vi "ESP301_StandAlone.vi"(0 "COM_PORT":string="COM13", 5 "stop":bool, 9 "SONDE_IN":bool) -> (3 "ESP301_ROT_MO":bool, 4 "ROT_mouvement":bool, 6 "ESP301_ROT_POS":dbl=3395.0 caption="Relacher pour \nmodifier TCS" format="%.2f", 8 "BRAS_OUT":bool, 10 "ESP301_BRAS_POS":dbl=3395.0 caption="Relacher pour \nmodifier TCS" format="%.2f", 14 "ESP301_BRAS_MO":bool, 15 "BRAS _mouvement":bool)   [LabVIEW 2019]
panel:
  in  "Reconnecter":bool
  in  "ROT_NORD_Value":dbl=120.0
  in  "BRAS_OUT_Value":dbl=40.0
  in  "BRAS_IN_Value":dbl=-6.0
  in  "BRAS_Target":dbl=30.0
  in  "BRAS_state":u16(ring) items=["Error"=6, "Stop"=5, "Out"=4, "In"=3, "Set"=2, "Home"=1, "Standby"=0]
  out "Comm":bool
  in  "ROT_Target":dbl=30.0
  in  "ROT_state":u16(ring) items=["Error"=6, "Stop"=4, "Nord"=3, "Set"=2, "Home"=1, "Standby"=0]
  in  "ESP301_BRAS_STOP":bool caption="À la cible"
  in  "ESP301_BRAS_SET":bool caption="À la cible"
  in  "ESP301_BRAS_OUT":bool caption="À la cible"
  in  "ESP301_BRAS_IN":bool caption="À la cible"
  in  "ESP301_BRAS_HOME":bool caption="À la cible"
  in  "ESP301_ROT_STOP":bool caption="À la cible"
  in  "ESP301_ROT_SET":bool caption="À la cible"
  in  "ESP301_ROT_NORD":bool caption="À la cible"
  in  "ESP301_ROT_HOME":bool caption="À la cible"
  # "Rotateur Pesto"
  # "Bras  Pesto"
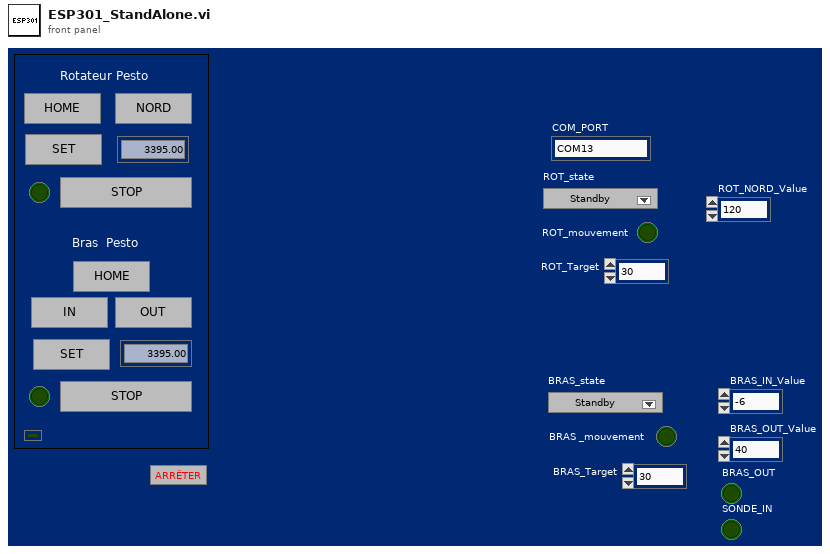
[diagram p1: front panel]
types:
  T1 = enum8{"Enabled", "Disabled", "Disabled and Grayed Out"}
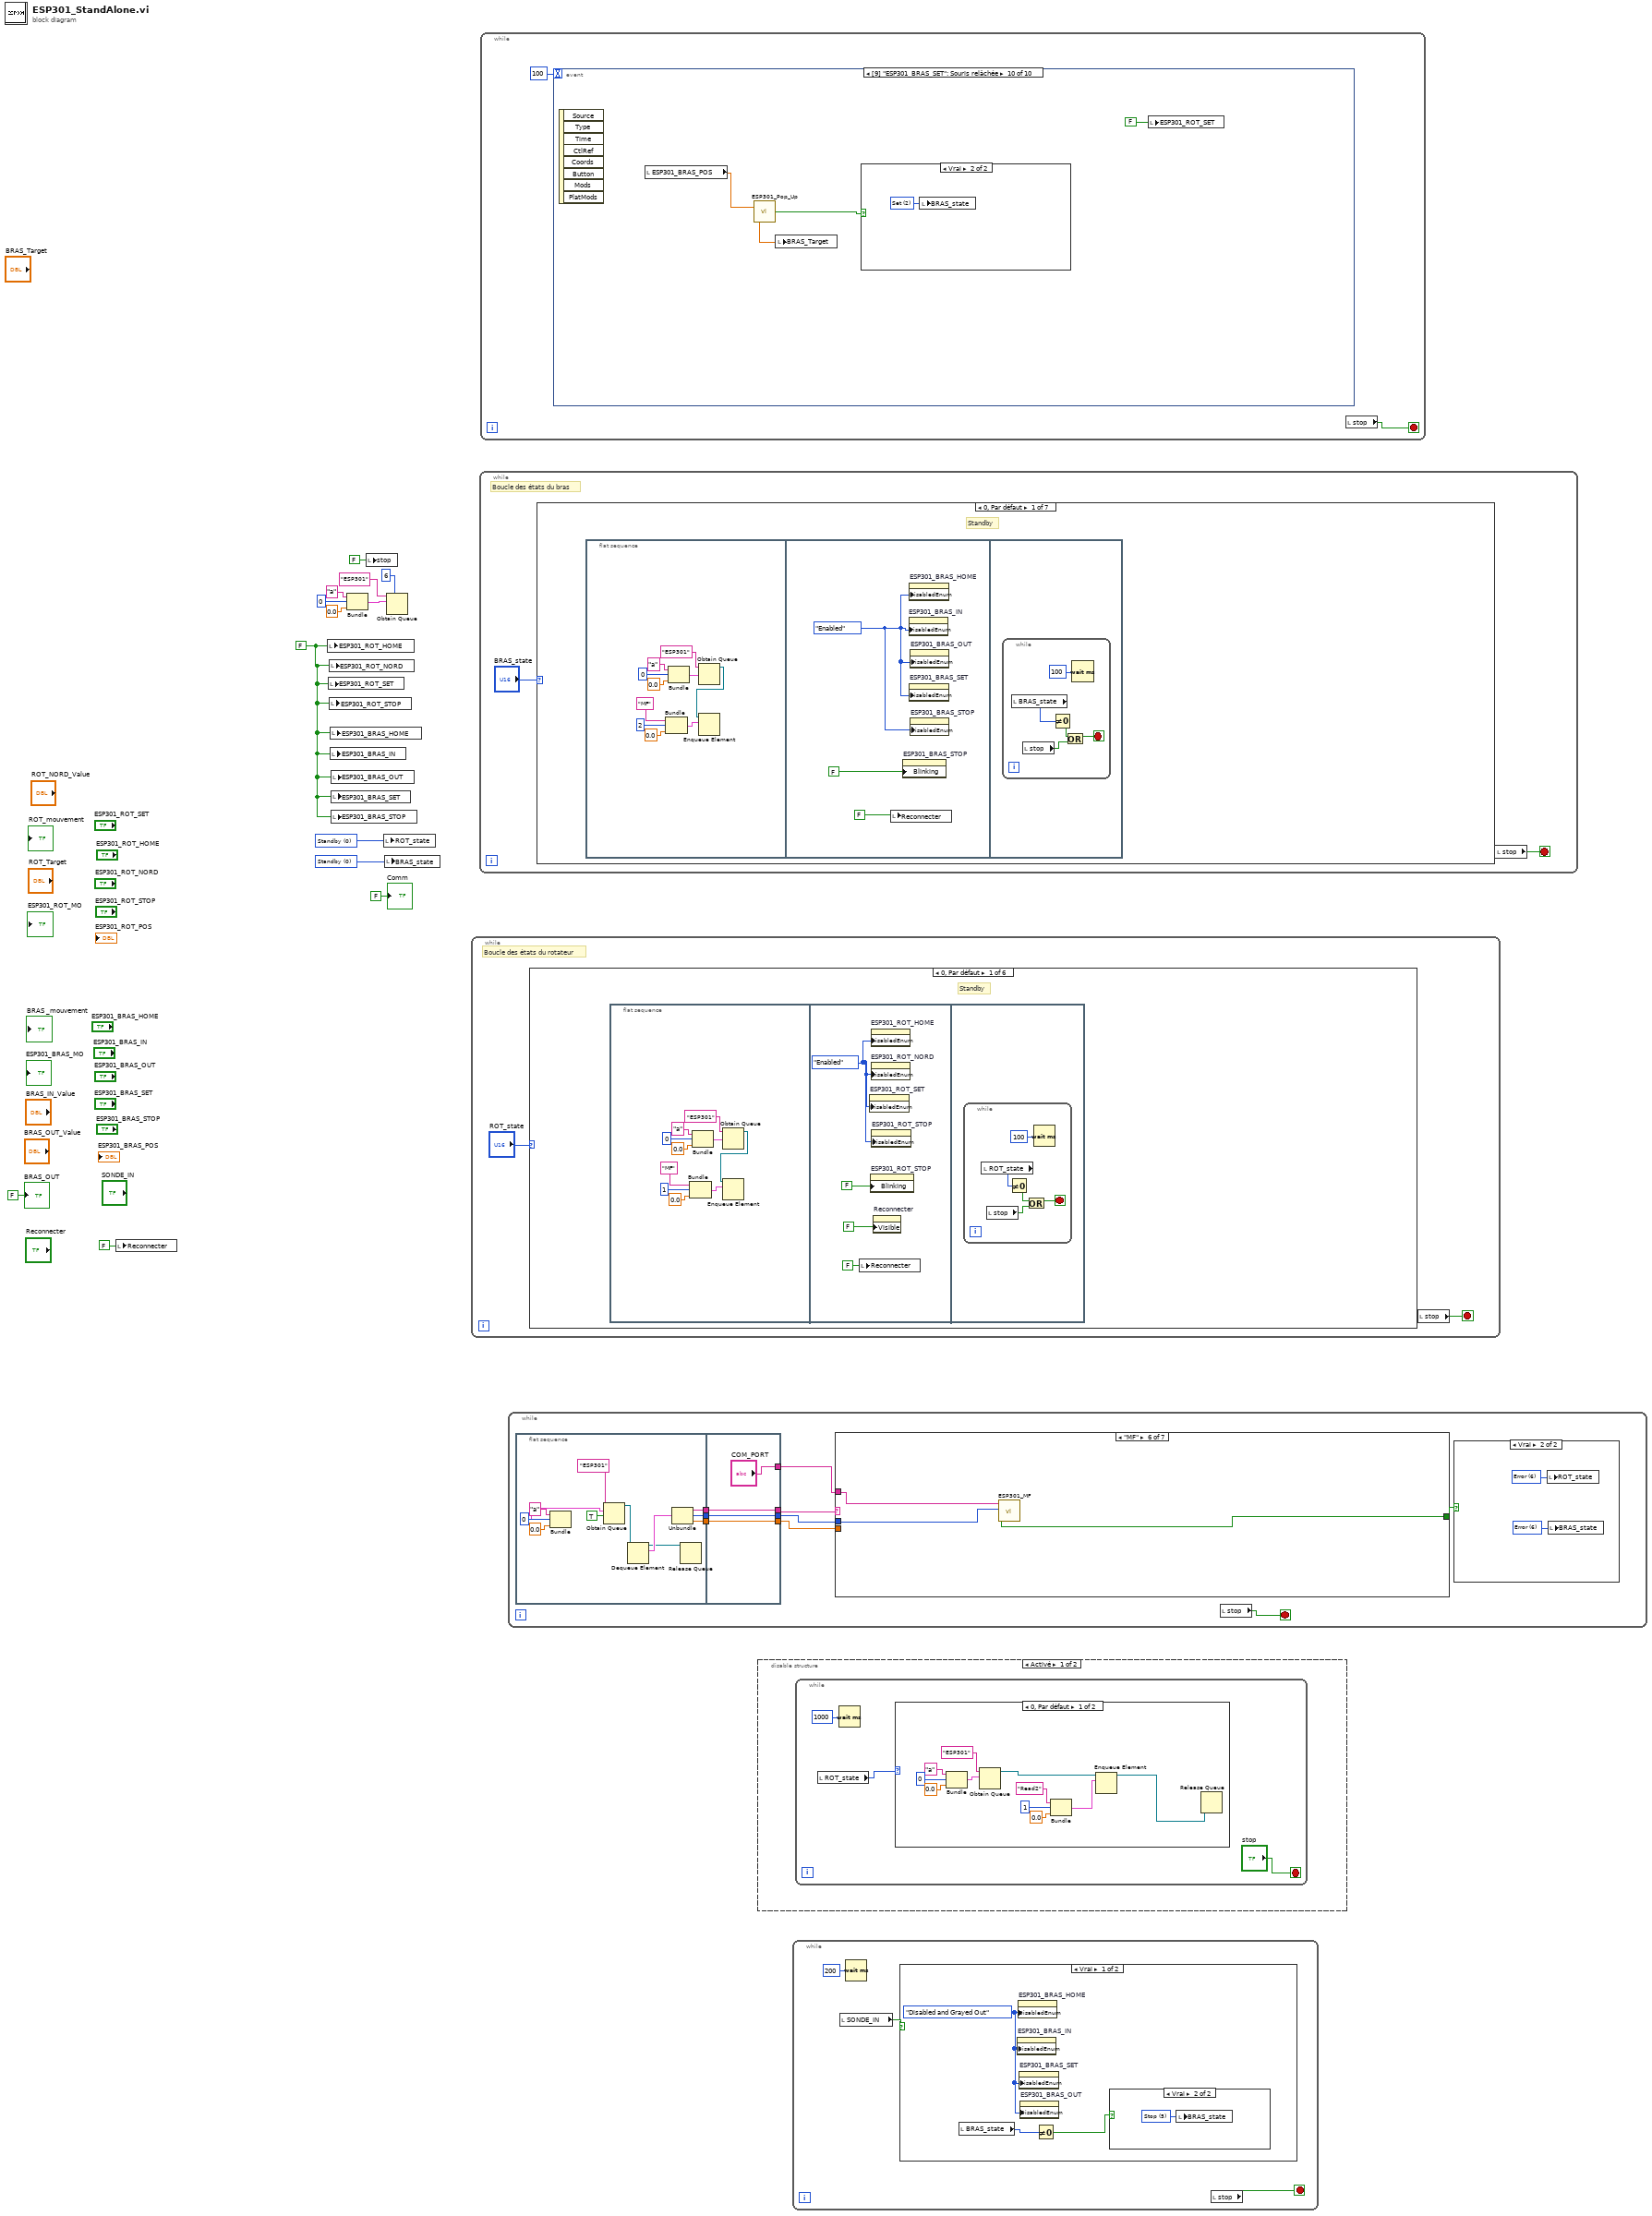
[diagram p0: block diagram]
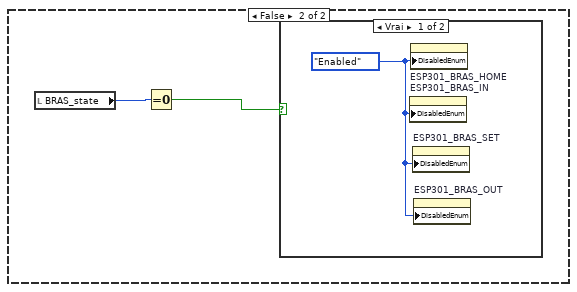
[diagram p3: hidden frame]
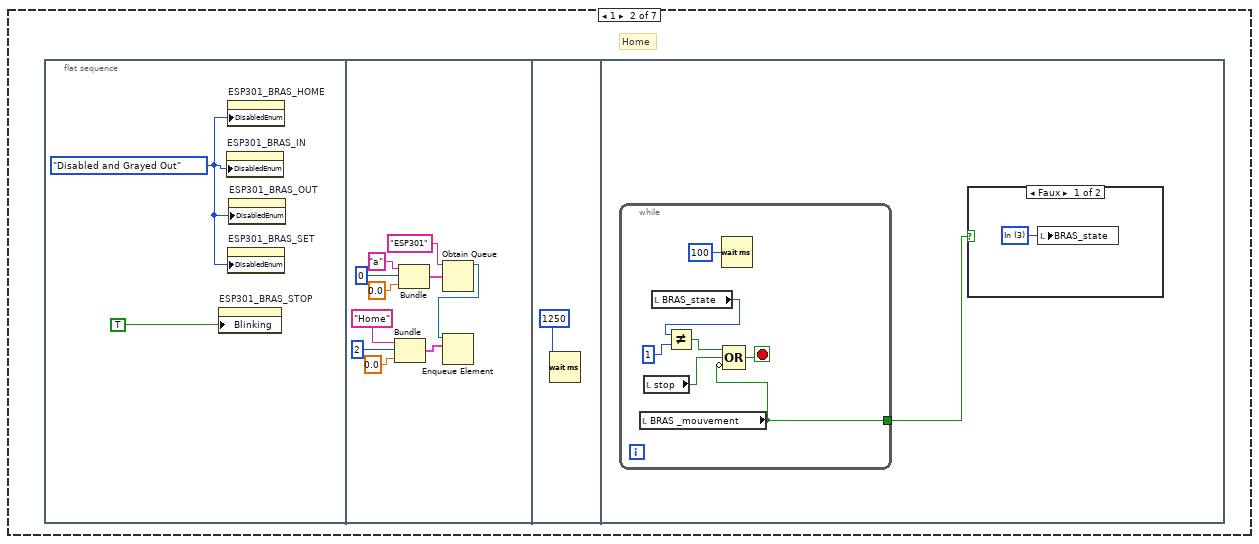
[diagram p5: hidden frame]
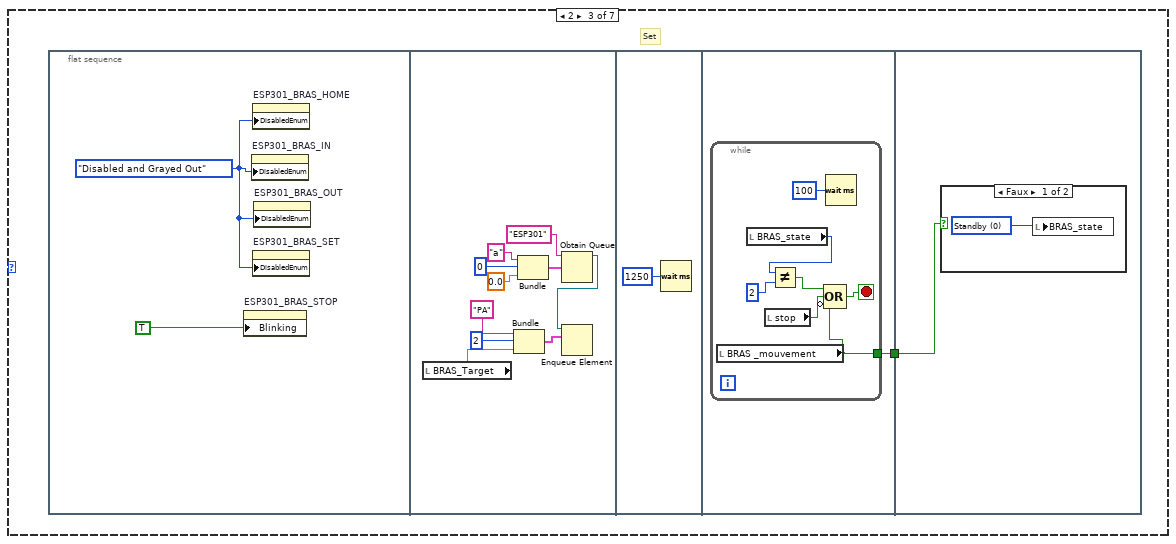
[diagram p7: hidden frame]
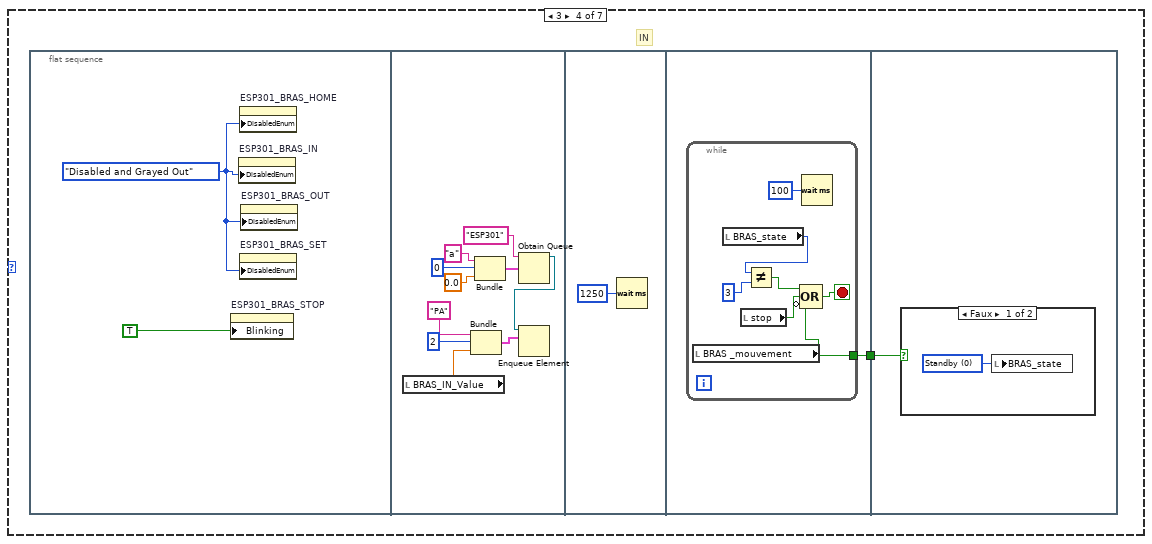
[diagram p9: hidden frame]
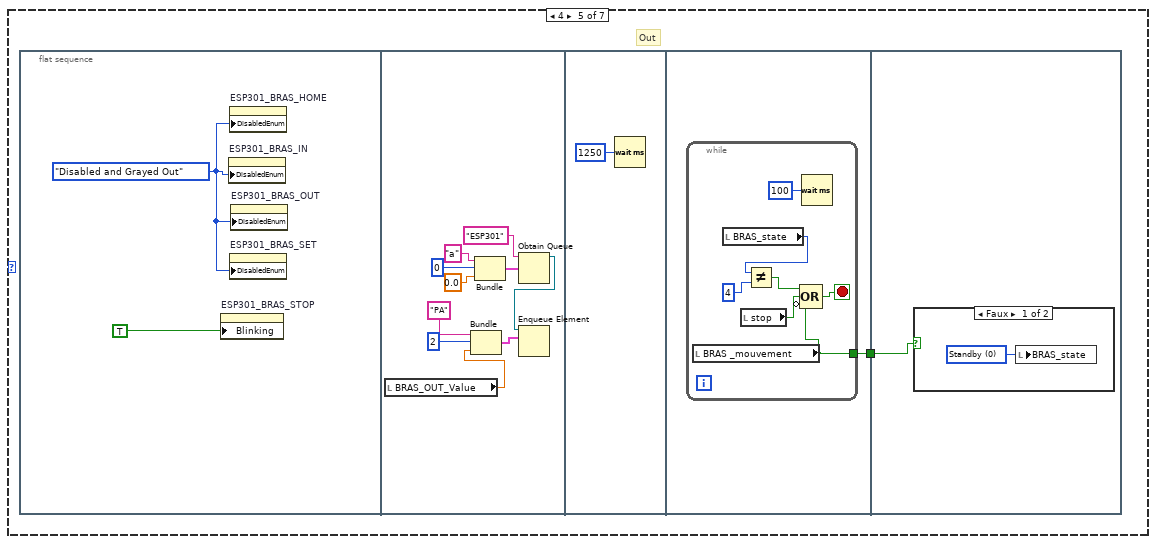
[diagram p11: hidden frame]
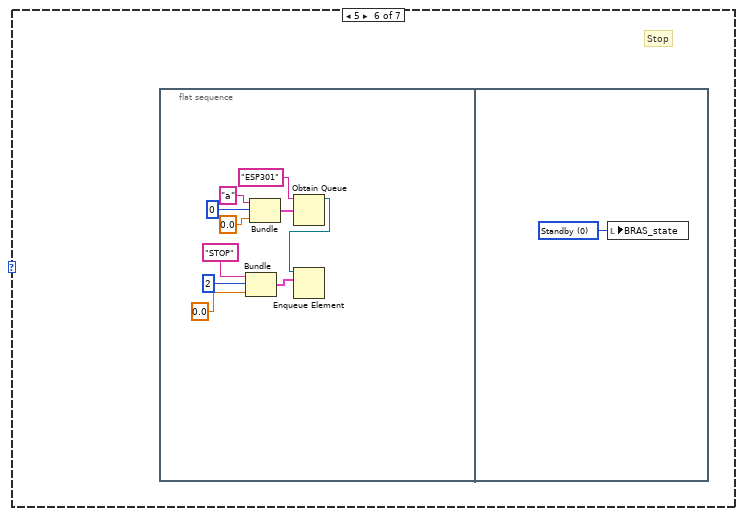
[diagram p13: hidden frame]
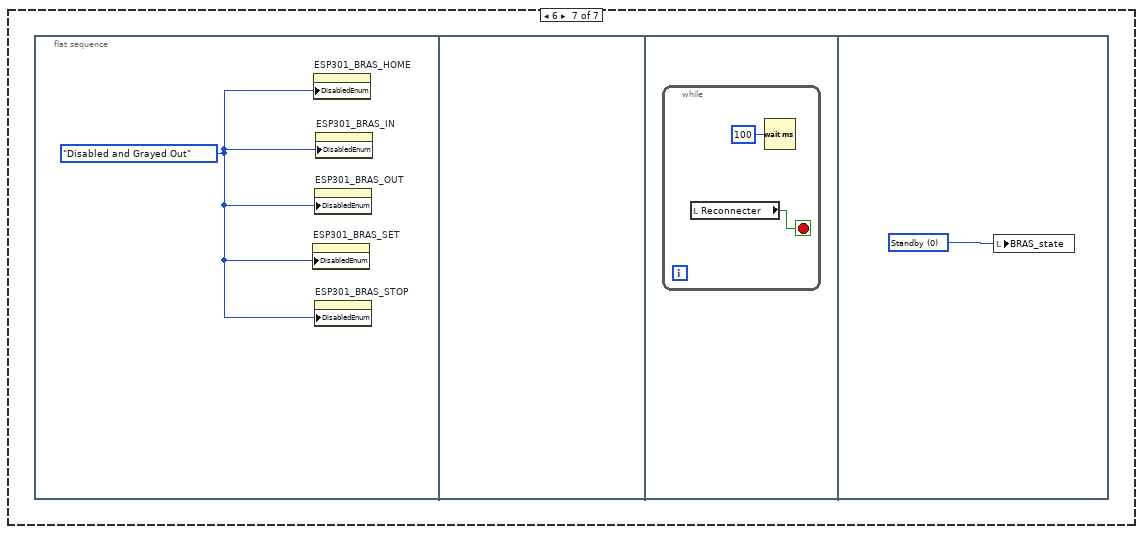
[diagram p14: hidden frame]
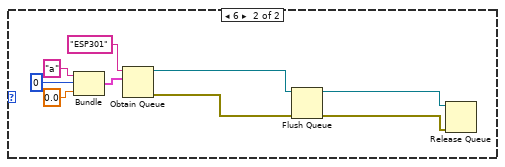
[diagram p15: hidden frame]
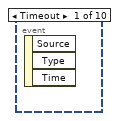
[diagram p17: hidden frame]
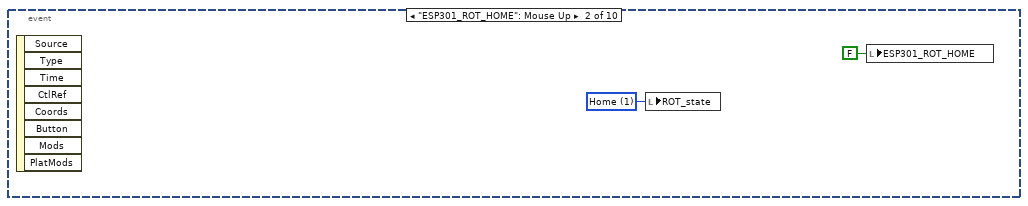
[diagram p18: hidden frame]
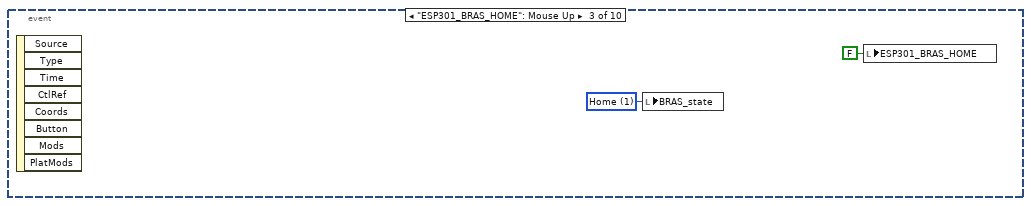
[diagram p19: hidden frame]
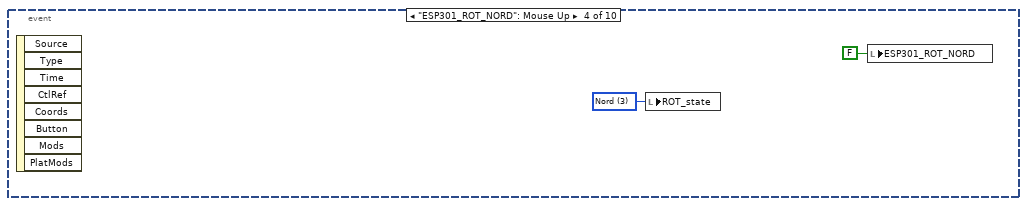
[diagram p20: hidden frame]
diagram:
  w4 = u16 0 items=["Stop"=4, "Nord"=3, "Set"=2, "Home"=1, "Standby"=0] ("BRAS_state")
  w5 = FALSE ("ESP301_ROT_HOME")
  w7 = u16 0 items=["Go"=2, "Home"=1, "Standby"=0] ("Rotateur_state")
  n1 = local write "Reconnecter"(FALSE ("Reconnecter")) -> ()
  n2 = local write "ESP301_ROT_HOME"(w5) -> ()
  n3 = local write "ESP301_ROT_SET"(w5) -> ()
  n4 = local write "ESP301_ROT_NORD"(w5) -> ()
  n5 = local write "ESP301_ROT_STOP"(w5) -> ()
  n6 = local write "ESP301_BRAS_HOME"(w5) -> ()
  n7 = local write "ESP301_BRAS_IN"(w5) -> ()
  n8 = local write "ESP301_BRAS_OUT"(w5) -> ()
  n9 = local write "ESP301_BRAS_SET"(w5) -> ()
  n10 = local write "ESP301_BRAS_STOP"(w5) -> ()
  n11 = Bundle("a", 0, 0.0) -> (w11:cluster{string, i32, dbl})  [unwired: 1 in]
  n12 = local write "stop"(FALSE ("stop")) -> ()
  n13 = local write "ROT_state"(w7) -> ()
  n14 = local write "BRAS_state"(w4) -> ()
  n15 = Obtain Queue(max queue size (-1, unlimited)=6 ("taille max de la file d'attente (-1, non limitée)"), name (unnamed)="ESP301" ("nom (aucun)"), element data type=w11) -> ()  [unwired: 2 in, 3 out]
  n16 = while {
    stop <- w15 stop-if-true
    # "Boucle des états du rotateur"
    n17 = case shown="0, Par défaut" "ROT_state" {
      frame 0, Default {
        # "Standby"
        n18 = flat-sequence {
          frame #0 {
            n19 = Bundle("MF", 1, 0.0) -> (w17:cluster{string, i32, dbl})  [unwired: 1 in]
            n20 = Bundle("a", 0, 0.0) -> (w23:cluster{string, i32, dbl})  [unwired: 1 in]
            n21 = Obtain Queue(name (unnamed)="ESP301" ("nom (aucun)"), element data type=w23) -> (queue out=w21:refnum<queue>)  [unwired: 3 in, 2 out]
            n22 = Enqueue Element(queue=w21, element=w17) -> ()  [unwired: 2 in, 3 out]
          }
          frame #1 {
            w27 = T1."Enabled" ("Désactivé")
            n23 = local write "Reconnecter"(FALSE ("Reconnecter")) -> ()
            n24 = property on="ESP301_ROT_SET" class="Bool (strict)"("DisabledEnum"=w27) -> ()  [unwired: 2 in, 2 out]
            n25 = property on="ESP301_ROT_STOP" class="Bool (strict)"("Blinking"=FALSE ("Clignotant")) -> ()  [unwired: 2 in, 2 out]
            n26 = property on="ESP301_ROT_HOME" class="Bool (strict)"("DisabledEnum"=w27) -> ()  [unwired: 2 in, 2 out]
            n27 = property on="ESP301_ROT_NORD" class="Bool (strict)"("DisabledEnum"=w27) -> ()  [unwired: 2 in, 2 out]
            n28 = property on="ESP301_ROT_STOP" class="Bool (strict)"("DisabledEnum"=w27) -> ()  [unwired: 2 in, 2 out]
            n29 = property on="Reconnecter" class="Bool (strict)"("Visible"=FALSE) -> ()  [unwired: 2 in, 2 out]
          }
          frame #2 {
            n30 = while {
              stop <- w32 stop-if-true
              n31 = local read "ROT_state"() -> (w34:u16)
              n32 = local read "stop"() -> (w31:bool)
              n33 = Not Equal To 0?(x=w34) -> (x != 0?=w30:bool)
              n34 = Or(x=w30, y=w31) -> (x .or. y?=w32:bool)
              n35 = Wait (ms)(milliseconds to wait=u32 100 ("attente (ms)")) -> ()  [unwired: 1 out]
            }
          }
        }
      }
      frame 1 {
        # "Home"
        n36 = flat-sequence {
          tunnel: [w49] -> w35
          tunnel: w35 -> [w57]
          frame #0 {
            w36 = T1."Disabled and Grayed Out" ("Désactivé")
            n37 = property on="ESP301_ROT_SET" class="Bool (strict)"("DisabledEnum"=w36) -> ()  [unwired: 2 in, 2 out]
            n38 = property on="ESP301_ROT_STOP" class="Bool (strict)"("Blinking"=TRUE ("Clignotant")) -> ()  [unwired: 2 in, 2 out]
            n39 = property on="ESP301_ROT_HOME" class="Bool (strict)"("DisabledEnum"=w36) -> ()  [unwired: 2 in, 2 out]
            n40 = property on="ESP301_ROT_NORD" class="Bool (strict)"("DisabledEnum"=w36) -> ()  [unwired: 2 in, 2 out]
          }
          frame #1 {
            n41 = local read "ROT_NORD_Value"() -> (w38:dbl)
            n42 = Bundle("Home", 1, "ROT_NORD_Value"=w38) -> (w40:cluster{string, i32, "ROT_NORD_Value":dbl})  [unwired: 1 in]
            n43 = Bundle("a", 0, 0.0) -> (w45:cluster{string, i32, dbl})  [unwired: 1 in]
            n44 = Obtain Queue(name (unnamed)="ESP301" ("nom (aucun)"), element data type=w45) -> (queue out=w43:refnum<queue>)  [unwired: 3 in, 2 out]
            n45 = Enqueue Element(queue=w43, element=w40) -> ()  [unwired: 2 in, 3 out]
          }
          frame #2 {
            n46 = Wait (ms)(milliseconds to wait=u32 1250 ("attente (ms)")) -> ()  [unwired: 1 out]
          }
          frame #3 {
            n47 = while {
              tunnel: [w50] -> w49
              stop <- w53 stop-if-true
              n48 = local read "stop"() -> (w51:bool)
              n49 = local read "ROT_state"() -> (w55:u16)
              n50 = local read "ROT_mouvement"() -> (w50:bool)
              n51 = Not Equal?(x=w55, y=u16 1) -> (x != y?=w52:bool)
              n52 = Wait (ms)(milliseconds to wait=u32 100 ("attente (ms)")) -> ()  [unwired: 1 out]
              n53 = Compound Arithmetic op=OR ("Opérateur arithmétique")(w52, w51, invert w50) -> (w53:bool)
            }
          }
          frame #4 {
            n54 = case shown="Faux" w57 {
              frame False {
                w58 = u16 3 items=["Stop"=4, "Nord"=3, "Set"=2, "Home"=1, "Standby"=0] ("ROT_state")
                n55 = local write "ROT_state"(w58) -> ()
              }
              frame True {
              }
            }
          }
        }
      }
      frame 2 {
        # "Set"
        n56 = flat-sequence {
          tunnel: [w73] -> w59
          tunnel: w59 -> [w81]
          frame #0 {
            w60 = T1."Disabled and Grayed Out" ("Désactivé")
            n57 = property on="ESP301_ROT_SET" class="Bool (strict)"("DisabledEnum"=w60) -> ()  [unwired: 2 in, 2 out]
            n58 = property on="ESP301_ROT_STOP" class="Bool (strict)"("Blinking"=TRUE ("Clignotant")) -> ()  [unwired: 2 in, 2 out]
            n59 = property on="ESP301_ROT_HOME" class="Bool (strict)"("DisabledEnum"=w60) -> ()  [unwired: 2 in, 2 out]
            n60 = property on="ESP301_ROT_NORD" class="Bool (strict)"("DisabledEnum"=w60) -> ()  [unwired: 2 in, 2 out]
          }
          frame #1 {
            n61 = local read "ROT_Target"() -> (w62:dbl)
            n62 = Bundle("PA", 1, "ROT_Target"=w62) -> (w64:cluster{string, i32, "ROT_Target":dbl})  [unwired: 1 in]
            n63 = Bundle("a", 0, 0.0) -> (w69:cluster{string, i32, dbl})  [unwired: 1 in]
            n64 = Obtain Queue(name (unnamed)="ESP301" ("nom (aucun)"), element data type=w69) -> (queue out=w67:refnum<queue>)  [unwired: 3 in, 2 out]
            n65 = Enqueue Element(queue=w67, element=w64) -> ()  [unwired: 2 in, 3 out]
          }
          frame #2 {
            n66 = Wait (ms)(milliseconds to wait=u32 1250 ("attente (ms)")) -> ()  [unwired: 1 out]
          }
          frame #3 {
            n67 = while {
              tunnel: [w74] -> w73
              stop <- w77 stop-if-true
              n68 = local read "ROT_mouvement"() -> (w74:bool)
              n69 = local read "ROT_state"() -> (w79:u16)
              n70 = local read "stop"() -> (w75:bool)
              n71 = Not Equal?(x=w79, y=u16 2) -> (x != y?=w76:bool)
              n72 = Compound Arithmetic op=OR ("Opérateur arithmétique")(w76, w75, invert w74) -> (w77:bool)
              n73 = Wait (ms)(milliseconds to wait=u32 100 ("attente (ms)")) -> ()  [unwired: 1 out]
            }
          }
          frame #4 {
            n74 = case shown="Faux" w81 {
              frame False {
                w82 = u16 0 items=["Nord"=3, "Go"=2, "Home"=1, "Standby"=0] ("ROT_state")
                n75 = local write "ROT_state"(w82) -> ()
              }
              frame True {
              }
            }
          }
        }
      }
      frame 3 {
        # "Nord"
        n76 = flat-sequence {
          tunnel: [w97] -> w83
          tunnel: w83 -> [w105]
          frame #0 {
            w84 = T1."Disabled and Grayed Out" ("Désactivé")
            n77 = property on="ESP301_ROT_SET" class="Bool (strict)"("DisabledEnum"=w84) -> ()  [unwired: 2 in, 2 out]
            n78 = property on="ESP301_ROT_STOP" class="Bool (strict)"("Blinking"=TRUE ("Clignotant")) -> ()  [unwired: 2 in, 2 out]
            n79 = property on="ESP301_ROT_HOME" class="Bool (strict)"("DisabledEnum"=w84) -> ()  [unwired: 2 in, 2 out]
            n80 = property on="ESP301_ROT_NORD" class="Bool (strict)"("DisabledEnum"=w84) -> ()  [unwired: 2 in, 2 out]
          }
          frame #1 {
            n81 = Bundle("PA", 1, 0.0) -> (w88:cluster{string, i32, dbl})  [unwired: 1 in]
            n82 = Bundle("a", 0, 0.0) -> (w93:cluster{string, i32, dbl})  [unwired: 1 in]
            n83 = Obtain Queue(name (unnamed)="ESP301" ("nom (aucun)"), element data type=w93) -> (queue out=w91:refnum<queue>)  [unwired: 3 in, 2 out]
            n84 = Enqueue Element(queue=w91, element=w88) -> ()  [unwired: 2 in, 3 out]
          }
          frame #2 {
            n85 = Wait (ms)(milliseconds to wait=u32 1250 ("attente (ms)")) -> ()  [unwired: 1 out]
          }
          frame #3 {
            n86 = while {
              tunnel: [w98] -> w97
              stop <- w101 stop-if-true
              n87 = local read "ROT_mouvement"() -> (w98:bool)
              n88 = local read "ROT_state"() -> (w103:u16)
              n89 = local read "stop"() -> (w99:bool)
              n90 = Not Equal?(x=w103, y=u16 3) -> (x != y?=w100:bool)
              n91 = Compound Arithmetic op=OR ("Opérateur arithmétique")(w100, w99, invert w98) -> (w101:bool)
              n92 = Wait (ms)(milliseconds to wait=u32 100 ("attente (ms)")) -> ()  [unwired: 1 out]
            }
          }
          frame #4 {
            n93 = case shown="Faux" w105 {
              frame False {
                w106 = u16 0 items=["Nord"=3, "Go"=2, "Home"=1, "Standby"=0] ("ROT_state")
                n94 = local write "ROT_state"(w106) -> ()
              }
              frame True {
              }
            }
          }
        }
      }
      frame 4 {
        # "Stop"
        n95 = flat-sequence {
          frame #0 {
            n96 = Bundle("STOP", 1, 0.0) -> (w109:cluster{string, i32, dbl})  [unwired: 1 in]
            n97 = Bundle("a", 0, 0.0) -> (w114:cluster{string, i32, dbl})  [unwired: 1 in]
            n98 = Obtain Queue(name (unnamed)="ESP301" ("nom (aucun)"), element data type=w114) -> (queue out=w112:refnum<queue>)  [unwired: 3 in, 2 out]
            n99 = Enqueue Element(queue=w112, element=w109) -> ()  [unwired: 2 in, 3 out]
          }
          frame #1 {
            w117 = u16 0 items=["Stop"=4, "Nord"=3, "Set"=2, "Home"=1, "Standby"=0] ("ROT_state")
            n100 = local write "ROT_state"(w117) -> ()
          }
        }
      }
      frame 6 {
        # "ERROR"
        n101 = flat-sequence {
          frame #0 {
            w119 = T1."Disabled and Grayed Out" ("Désactivé")
            n102 = property on="ESP301_ROT_SET" class="Bool (strict)"("DisabledEnum"=w119) -> ()  [unwired: 2 in, 2 out]
            n103 = property on="ESP301_ROT_HOME" class="Bool (strict)"("DisabledEnum"=w119) -> ()  [unwired: 2 in, 2 out]
            n104 = property on="ESP301_ROT_NORD" class="Bool (strict)"("DisabledEnum"=w119) -> ()  [unwired: 2 in, 2 out]
            n105 = property on="ESP301_ROT_STOP" class="Bool (strict)"("DisabledEnum"=w119) -> ()  [unwired: 2 in, 2 out]
            n106 = property on="Reconnecter" class="Bool (strict)"("Visible"=TRUE) -> ()  [unwired: 2 in, 2 out]
          }
          frame #1 {
          }
          frame #2 {
            n107 = while {
              stop <- w120 stop-if-true
              n108 = local read "Reconnecter"() -> (w120:bool)
              n109 = Wait (ms)(milliseconds to wait=u32 100 ("attente (ms)")) -> ()  [unwired: 1 out]
            }
          }
          frame #3 {
            w122 = u16 0 items=["Error"=6, "Stop"=4, "Nord"=3, "Set"=2, "Home"=1, "Standby"=0] ("ROT_state")
            n110 = local write "ROT_state"(w122) -> ()
          }
        }
      }
    }
    n111 = local read "stop"() -> (w15:bool)
  }
  n112 = while {
    stop <- w124 stop-if-true
    # "Boucle des états du bras"
    n113 = case shown="0, Par défaut" "BRAS_state" {
      frame 0, Default {
        # "Standby"
        n114 = flat-sequence {
          frame #0 {
            n115 = Bundle("MF", 2, 0.0) -> (w126:cluster{string, i32, dbl})  [unwired: 1 in]
            n116 = Bundle("a", 0, 0.0) -> (w132:cluster{string, i32, dbl})  [unwired: 1 in]
            n117 = Obtain Queue(name (unnamed)="ESP301" ("nom (aucun)"), element data type=w132) -> (queue out=w130:refnum<queue>)  [unwired: 3 in, 2 out]
            n118 = Enqueue Element(queue=w130, element=w126) -> ()  [unwired: 2 in, 3 out]
          }
          frame #1 {
            w135 = T1."Enabled" ("Désactivé")
            n119 = local write "Reconnecter"(FALSE ("Reconnecter")) -> ()
            n120 = property on="ESP301_BRAS_STOP" class="Bool (strict)"("Blinking"=FALSE ("Clignotant")) -> ()  [unwired: 2 in, 2 out]
            n121 = property on="ESP301_BRAS_IN" class="Bool (strict)"("DisabledEnum"=w135) -> ()  [unwired: 2 in, 2 out]
            n122 = property on="ESP301_BRAS_HOME" class="Bool (strict)"("DisabledEnum"=w135) -> ()  [unwired: 2 in, 2 out]
            n123 = property on="ESP301_BRAS_SET" class="Bool (strict)"("DisabledEnum"=w135) -> ()  [unwired: 2 in, 2 out]
            n124 = property on="ESP301_BRAS_OUT" class="Bool (strict)"("DisabledEnum"=w135) -> ()  [unwired: 2 in, 2 out]
            n125 = property on="ESP301_BRAS_STOP" class="Bool (strict)"("DisabledEnum"=w135) -> ()  [unwired: 2 in, 2 out]
          }
          frame #2 {
            n126 = while {
              stop <- w141 stop-if-true
              n127 = local read "BRAS_state"() -> (w138:u16)
              n128 = local read "stop"() -> (w139:bool)
              n129 = Not Equal To 0?(x=w138) -> (x != 0?=w140:bool)
              n130 = Or(x=w140, y=w139) -> (x .or. y?=w141:bool)
              n131 = Wait (ms)(milliseconds to wait=u32 100 ("attente (ms)")) -> ()  [unwired: 1 out]
            }
          }
        }
      }
      frame 1 {
        # "Home"
        n132 = flat-sequence {
          frame #0 {
            w144 = T1."Disabled and Grayed Out" ("Désactivé")
            n133 = property on="ESP301_BRAS_STOP" class="Bool (strict)"("Blinking"=TRUE ("Clignotant")) -> ()  [unwired: 2 in, 2 out]
            n134 = property on="ESP301_BRAS_IN" class="Bool (strict)"("DisabledEnum"=w144) -> ()  [unwired: 2 in, 2 out]
            n135 = property on="ESP301_BRAS_HOME" class="Bool (strict)"("DisabledEnum"=w144) -> ()  [unwired: 2 in, 2 out]
            n136 = property on="ESP301_BRAS_SET" class="Bool (strict)"("DisabledEnum"=w144) -> ()  [unwired: 2 in, 2 out]
            n137 = property on="ESP301_BRAS_OUT" class="Bool (strict)"("DisabledEnum"=w144) -> ()  [unwired: 2 in, 2 out]
          }
          frame #1 {
            n138 = Bundle("Home", 2, 0.0) -> (w146:cluster{string, i32, dbl})  [unwired: 1 in]
            n139 = Bundle("a", 0, 0.0) -> (w152:cluster{string, i32, dbl})  [unwired: 1 in]
            n140 = Obtain Queue(name (unnamed)="ESP301" ("nom (aucun)"), element data type=w152) -> (queue out=w150:refnum<queue>)  [unwired: 3 in, 2 out]
            n141 = Enqueue Element(queue=w150, element=w146) -> ()  [unwired: 2 in, 3 out]
          }
          frame #2 {
            n142 = Wait (ms)(milliseconds to wait=u32 1250 ("attente (ms)")) -> ()  [unwired: 1 out]
          }
          frame #3 {
            n143 = while {
              tunnel: [w158] -> w156
              stop <- w162 stop-if-true
              n144 = local read "BRAS _mouvement"() -> (w158:bool)
              n145 = local read "stop"() -> (w159:bool)
              n146 = local read "BRAS_state"() -> (w160:u16)
              n147 = Not Equal?(x=w160, y=u16 1) -> (x != y?=w161:bool)
              n148 = Wait (ms)(milliseconds to wait=u32 100 ("attente (ms)")) -> ()  [unwired: 1 out]
              n149 = Compound Arithmetic op=OR ("Opérateur arithmétique")(w161, w159, invert w158) -> (w162:bool)
            }
            n150 = case shown="Faux" w156 {
              frame False {
                w157 = u16 3 items=["Stop"=5, "Out"=4, "In"=3, "Set"=2, "Home"=1, "Standby"=0] ("BRAS_state")
                n151 = local write "BRAS_state"(w157) -> ()
              }
              frame True {
              }
            }
          }
        }
      }
      frame 2 {
        # "Set"
        n152 = flat-sequence {
          tunnel: [w179] -> w165
          tunnel: w165 -> [w187]
          frame #0 {
            w167 = T1."Disabled and Grayed Out" ("Désactivé")
            n153 = property on="ESP301_BRAS_STOP" class="Bool (strict)"("Blinking"=TRUE ("Clignotant")) -> ()  [unwired: 2 in, 2 out]
            n154 = property on="ESP301_BRAS_IN" class="Bool (strict)"("DisabledEnum"=w167) -> ()  [unwired: 2 in, 2 out]
            n155 = property on="ESP301_BRAS_HOME" class="Bool (strict)"("DisabledEnum"=w167) -> ()  [unwired: 2 in, 2 out]
            n156 = property on="ESP301_BRAS_SET" class="Bool (strict)"("DisabledEnum"=w167) -> ()  [unwired: 2 in, 2 out]
            n157 = property on="ESP301_BRAS_OUT" class="Bool (strict)"("DisabledEnum"=w167) -> ()  [unwired: 2 in, 2 out]
          }
          frame #1 {
            n158 = local read "BRAS_Target"() -> (w168:dbl)
            n159 = Bundle("PA", 2, "BRAS_Target"=w168) -> (w170:cluster{string, i32, "BRAS_Target":dbl})  [unwired: 1 in]
            n160 = Bundle("a", 0, 0.0) -> (w175:cluster{string, i32, dbl})  [unwired: 1 in]
            n161 = Obtain Queue(name (unnamed)="ESP301" ("nom (aucun)"), element data type=w175) -> (queue out=w173:refnum<queue>)  [unwired: 3 in, 2 out]
            n162 = Enqueue Element(queue=w173, element=w170) -> ()  [unwired: 2 in, 3 out]
          }
          frame #2 {
            n163 = Wait (ms)(milliseconds to wait=u32 1250 ("attente (ms)")) -> ()  [unwired: 1 out]
          }
          frame #3 {
            n164 = while {
              tunnel: [w180] -> w179
              stop <- w183 stop-if-true
              n165 = local read "BRAS _mouvement"() -> (w180:bool)
              n166 = local read "BRAS_state"() -> (w185:u16)
              n167 = local read "stop"() -> (w181:bool)
              n168 = Not Equal?(x=w185, y=u16 2) -> (x != y?=w182:bool)
              n169 = Compound Arithmetic op=OR ("Opérateur arithmétique")(w182, w181, invert w180) -> (w183:bool)
              n170 = Wait (ms)(milliseconds to wait=u32 100 ("attente (ms)")) -> ()  [unwired: 1 out]
            }
          }
          frame #4 {
            n171 = case shown="Faux" w187 {
              frame False {
                w188 = u16 0 items=["Stop"=5, "Out"=4, "In"=3, "Set"=2, "Home"=1, "Standby"=0] ("BRAS_state")
                n172 = local write "BRAS_state"(w188) -> ()
              }
              frame True {
              }
            }
          }
        }
      }
      frame 3 {
        # "IN"
        n173 = flat-sequence {
          tunnel: [w203] -> w189
          tunnel: w189 -> [w211]
          frame #0 {
            w191 = T1."Disabled and Grayed Out" ("Désactivé")
            n174 = property on="ESP301_BRAS_STOP" class="Bool (strict)"("Blinking"=TRUE ("Clignotant")) -> ()  [unwired: 2 in, 2 out]
            n175 = property on="ESP301_BRAS_IN" class="Bool (strict)"("DisabledEnum"=w191) -> ()  [unwired: 2 in, 2 out]
            n176 = property on="ESP301_BRAS_HOME" class="Bool (strict)"("DisabledEnum"=w191) -> ()  [unwired: 2 in, 2 out]
            n177 = property on="ESP301_BRAS_SET" class="Bool (strict)"("DisabledEnum"=w191) -> ()  [unwired: 2 in, 2 out]
            n178 = property on="ESP301_BRAS_OUT" class="Bool (strict)"("DisabledEnum"=w191) -> ()  [unwired: 2 in, 2 out]
          }
          frame #1 {
            n179 = local read "BRAS_IN_Value"() -> (w192:dbl)
            n180 = Bundle("PA", 2, "BRAS_IN_Value"=w192) -> (w194:cluster{string, i32, "BRAS_IN_Value":dbl})  [unwired: 1 in]
            n181 = Bundle("a", 0, 0.0) -> (w199:cluster{string, i32, dbl})  [unwired: 1 in]
            n182 = Obtain Queue(name (unnamed)="ESP301" ("nom (aucun)"), element data type=w199) -> (queue out=w197:refnum<queue>)  [unwired: 3 in, 2 out]
            n183 = Enqueue Element(queue=w197, element=w194) -> ()  [unwired: 2 in, 3 out]
          }
          frame #2 {
            n184 = Wait (ms)(milliseconds to wait=u32 1250 ("attente (ms)")) -> ()  [unwired: 1 out]
          }
          frame #3 {
            n185 = while {
              tunnel: [w204] -> w203
              stop <- w207 stop-if-true
              n186 = local read "BRAS _mouvement"() -> (w204:bool)
              n187 = local read "BRAS_state"() -> (w209:u16)
              n188 = local read "stop"() -> (w205:bool)
              n189 = Not Equal?(x=w209, y=u16 3) -> (x != y?=w206:bool)
              n190 = Compound Arithmetic op=OR ("Opérateur arithmétique")(w206, w205, invert w204) -> (w207:bool)
              n191 = Wait (ms)(milliseconds to wait=u32 100 ("attente (ms)")) -> ()  [unwired: 1 out]
            }
          }
          frame #4 {
            n192 = case shown="Faux" w211 {
              frame False {
                w212 = u16 0 items=["Stop"=5, "Out"=4, "In"=3, "Set"=2, "Home"=1, "Standby"=0] ("BRAS_state")
                n193 = local write "BRAS_state"(w212) -> ()
              }
              frame True {
              }
            }
          }
        }
      }
      frame 4 {
        # "Out"
        n194 = flat-sequence {
          tunnel: [w227] -> w213
          tunnel: w213 -> [w235]
          frame #0 {
            w215 = T1."Disabled and Grayed Out" ("Désactivé")
            n195 = property on="ESP301_BRAS_STOP" class="Bool (strict)"("Blinking"=TRUE ("Clignotant")) -> ()  [unwired: 2 in, 2 out]
            n196 = property on="ESP301_BRAS_IN" class="Bool (strict)"("DisabledEnum"=w215) -> ()  [unwired: 2 in, 2 out]
            n197 = property on="ESP301_BRAS_HOME" class="Bool (strict)"("DisabledEnum"=w215) -> ()  [unwired: 2 in, 2 out]
            n198 = property on="ESP301_BRAS_SET" class="Bool (strict)"("DisabledEnum"=w215) -> ()  [unwired: 2 in, 2 out]
            n199 = property on="ESP301_BRAS_OUT" class="Bool (strict)"("DisabledEnum"=w215) -> ()  [unwired: 2 in, 2 out]
          }
          frame #1 {
            n200 = local read "BRAS_OUT_Value"() -> (w216:dbl)
            n201 = Bundle("PA", 2, "BRAS_OUT_Value"=w216) -> (w218:cluster{string, i32, "BRAS_OUT_Value":dbl})  [unwired: 1 in]
            n202 = Bundle("a", 0, 0.0) -> (w223:cluster{string, i32, dbl})  [unwired: 1 in]
            n203 = Obtain Queue(name (unnamed)="ESP301" ("nom (aucun)"), element data type=w223) -> (queue out=w221:refnum<queue>)  [unwired: 3 in, 2 out]
            n204 = Enqueue Element(queue=w221, element=w218) -> ()  [unwired: 2 in, 3 out]
          }
          frame #2 {
            n205 = Wait (ms)(milliseconds to wait=u32 1250 ("attente (ms)")) -> ()  [unwired: 1 out]
          }
          frame #3 {
            n206 = while {
              tunnel: [w228] -> w227
              stop <- w231 stop-if-true
              n207 = local read "BRAS _mouvement"() -> (w228:bool)
              n208 = local read "BRAS_state"() -> (w233:u16)
              n209 = local read "stop"() -> (w229:bool)
              n210 = Not Equal?(x=w233, y=u16 4) -> (x != y?=w230:bool)
              n211 = Compound Arithmetic op=OR ("Opérateur arithmétique")(w230, w229, invert w228) -> (w231:bool)
              n212 = Wait (ms)(milliseconds to wait=u32 100 ("attente (ms)")) -> ()  [unwired: 1 out]
            }
          }
          frame #4 {
            n213 = case shown="Faux" w235 {
              frame False {
                w236 = u16 0 items=["Stop"=5, "Out"=4, "In"=3, "Set"=2, "Home"=1, "Standby"=0] ("BRAS_state")
                n214 = local write "BRAS_state"(w236) -> ()
              }
              frame True {
              }
            }
          }
        }
      }
      frame 5 {
        # "Stop"
        n215 = flat-sequence {
          frame #0 {
            n216 = Bundle("STOP", 2, 0.0) -> (w239:cluster{string, i32, dbl})  [unwired: 1 in]
            n217 = Bundle("a", 0, 0.0) -> (w244:cluster{string, i32, dbl})  [unwired: 1 in]
            n218 = Obtain Queue(name (unnamed)="ESP301" ("nom (aucun)"), element data type=w244) -> (queue out=w242:refnum<queue>)  [unwired: 3 in, 2 out]
            n219 = Enqueue Element(queue=w242, element=w239) -> ()  [unwired: 2 in, 3 out]
          }
          frame #1 {
            w247 = u16 0 items=["Stop"=5, "Out"=4, "In"=3, "Set"=2, "Home"=1, "Standby"=0] ("BRAS_state")
            n220 = local write "BRAS_state"(w247) -> ()
          }
        }
      }
      frame 6 {
        n221 = flat-sequence {
          frame #0 {
            w248 = T1."Disabled and Grayed Out" ("Désactivé")
            n222 = property on="ESP301_BRAS_SET" class="Bool (strict)"("DisabledEnum"=w248) -> ()  [unwired: 2 in, 2 out]
            n223 = property on="ESP301_BRAS_HOME" class="Bool (strict)"("DisabledEnum"=w248) -> ()  [unwired: 2 in, 2 out]
            n224 = property on="ESP301_BRAS_OUT" class="Bool (strict)"("DisabledEnum"=w248) -> ()  [unwired: 2 in, 2 out]
            n225 = property on="ESP301_BRAS_STOP" class="Bool (strict)"("DisabledEnum"=w248) -> ()  [unwired: 2 in, 2 out]
            n226 = property on="ESP301_BRAS_IN" class="Bool (strict)"("DisabledEnum"=w248) -> ()  [unwired: 2 in, 2 out]
          }
          frame #1 {
          }
          frame #2 {
            n227 = while {
              stop <- w249 stop-if-true
              n228 = local read "Reconnecter"() -> (w249:bool)
              n229 = Wait (ms)(milliseconds to wait=u32 100 ("attente (ms)")) -> ()  [unwired: 1 out]
            }
          }
          frame #3 {
            w251 = u16 0 items=["Error"=6, "Stop"=5, "Out"=4, "In"=3, "Set"=2, "Home"=1, "Standby"=0] ("BRAS_state")
            n230 = local write "BRAS_state"(w251) -> ()
          }
        }
      }
    }
    n231 = local read "stop"() -> (w124:bool)
  }
  n232 = while {
    stop <- w253 stop-if-true
    n233 = event shown="[9] \"ESP301_BRAS_SET\": Souris relâchée" {
      selector: _ -> [_ _ _ _ _ _ _ _ _ _]
      dyn-events: _ -> [_ _ _ _ _ _ _ _ _ _]
      timeout: 100 -> [_ _ _ _ _ _ _ _ _ _]
      event Timeout {
        n234 = event-data() -> ()  [unwired: 1 in, 3 out]
      }
      event "ESP301_ROT_HOME": Mouse Up {
        w254 = u16 1 items=["Nord"=3, "Go"=2, "Home"=1, "Standby"=0] ("ROT_state")
        n235 = event-data() -> ()  [unwired: 1 in, 8 out]
        n236 = local write "ROT_state"(w254) -> ()
        n237 = local write "ESP301_ROT_HOME"(FALSE ("ESP301_ROT_HOME")) -> ()
      }
      event "ESP301_BRAS_HOME": Mouse Up {
        w256 = u16 1 items=["Nord"=3, "Go"=2, "Home"=1, "Standby"=0] ("ROT_state")
        n238 = event-data() -> ()  [unwired: 1 in, 8 out]
        n239 = local write "BRAS_state"(w256) -> ()
        n240 = local write "ESP301_BRAS_HOME"(FALSE ("ESP301_ROT_HOME")) -> ()
      }
      event "ESP301_ROT_NORD": Mouse Up {
        w258 = u16 3 items=["Nord"=3, "Go"=2, "Home"=1, "Standby"=0] ("ROT_state")
        n241 = event-data() -> ()  [unwired: 1 in, 8 out]
        n242 = local write "ROT_state"(w258) -> ()
        n243 = local write "ESP301_ROT_NORD"(FALSE ("ESP301_ROT_HOME")) -> ()
      }
      event "ESP301_BRAS_IN": Mouse Up {
        w260 = u16 3 items=["Stop"=5, "Out"=4, "In"=3, "Set"=2, "Home"=1, "Standby"=0] ("BRAS_state")
        n244 = event-data() -> ()  [unwired: 1 in, 8 out]
        n245 = local write "BRAS_state"(w260) -> ()
        n246 = local write "ESP301_BRAS_IN"(FALSE ("ESP301_ROT_HOME")) -> ()
      }
      event "ESP301_BRAS_OUT": Mouse Up {
        w262 = u16 4 items=["Stop"=5, "Out"=4, "In"=3, "Set"=2, "Home"=1, "Standby"=0] ("BRAS_state")
        n247 = event-data() -> ()  [unwired: 1 in, 8 out]
        n248 = local write "BRAS_state"(w262) -> ()
        n249 = local write "ESP301_BRAS_OUT"(FALSE ("ESP301_ROT_HOME")) -> ()
      }
      event "ESP301_ROT_STOP": Mouse Up {
        w264 = u16 4 items=["Stop"=4, "Nord"=3, "Set"=2, "Home"=1, "Standby"=0] ("ROT_state")
        n250 = event-data() -> ()  [unwired: 1 in, 8 out]
        n251 = local write "ROT_state"(w264) -> ()
        n252 = local write "ESP301_ROT_STOP"(FALSE ("ESP301_ROT_HOME")) -> ()
      }
      event "ESP301_BRAS_STOP": Mouse Up {
        w266 = u16 5 items=["Stop"=5, "Out"=4, "In"=3, "Set"=2, "Home"=1, "Standby"=0] ("BRAS_state")
        n253 = event-data() -> ()  [unwired: 1 in, 8 out]
        n254 = local write "BRAS_state"(w266) -> ()
        n255 = local write "ESP301_BRAS_STOP"(FALSE ("ESP301_ROT_HOME")) -> ()
      }
      event "ESP301_ROT_SET": Mouse Up {
        n256 = event-data() -> ()  [unwired: 1 in, 8 out]
        n257 = local read "ESP301_ROT_POS"() -> (w269:dbl)
        n258 = call "ESP301_Pop_Up.vi"("Rot.In"=w269) -> ("DONE"=w270:bool, "Rot.Out"=w268:dbl)
        n259 = local write "ROT_Target"(w268) -> ()
        n260 = case shown="Vrai" w270 {
          frame False {
          }
          frame True {
            w272 = u16 2 items=["Stop"=4, "Nord"=3, "Set"=2, "Home"=1, "Standby"=0] ("ROT_state")
            n261 = local write "ROT_state"(w272) -> ()
          }
        }
        n262 = local write "ESP301_ROT_SET"(FALSE ("ESP301_ROT_HOME")) -> ()
      }
      event "ESP301_BRAS_SET": Mouse Up {
        n263 = event-data() -> ()  [unwired: 1 in, 8 out]
        n264 = local read "ESP301_BRAS_POS"() -> (w274:dbl)
        n265 = call "ESP301_Pop_Up.vi"("Rot.In"=w274) -> ("DONE"=w275:bool, "Rot.Out"=w273:dbl)
        n266 = local write "BRAS_Target"(w273) -> ()
        n267 = case shown="Vrai" w275 {
          frame False {
          }
          frame True {
            w277 = u16 2 items=["Stop"=5, "Out"=4, "In"=3, "Set"=2, "Home"=1, "Standby"=0] ("BRAS_state")
            n268 = local write "BRAS_state"(w277) -> ()
          }
        }
        n269 = local write "ESP301_ROT_SET"(FALSE ("ESP301_ROT_HOME")) -> ()
      }
    }
    n270 = local read "stop"() -> (w253:bool)
  }
  n271 = while {
    stop <- w284 stop-if-true
    n272 = flat-sequence {
      tunnel: [w297] -> w281
      tunnel: [w296] -> w280
      tunnel: [w287] -> w279
      tunnel: [w300] -> w283
      tunnel: [w301] -> w285
      tunnel: [w302] -> w286
      tunnel: w281 -> [w302]
      tunnel: w280 -> [w301]
      tunnel: w279 -> [w300]
      tunnel: ["COM_PORT"] -> w278
      frame #0 {
        n273 = Bundle("a", 0, 0.0) -> (w288:cluster{string, i32, dbl})  [unwired: 1 in]
        n274 = Obtain Queue(name (unnamed)="ESP301" ("nom (aucun)"), element data type=w288, create if not found? (T)=TRUE ("créer si introuvable ? (V)")) -> (queue out=w294:refnum<queue>)  [unwired: 2 in, 2 out]
        n275 = Dequeue Element(queue=w294) -> (queue out=w295:refnum<queue>, element=w298:cluster{string, i32, dbl})  [unwired: 2 in, 2 out]
        n276 = Unbundle(w298) -> (w297:string, w296:i32, w287:dbl)
        n277 = Release Queue(queue=w295) -> ()  [unwired: 2 in, 3 out]
      }
      frame #1 {
      }
    }
    n278 = case shown="\"MF\"" w286 {
      tunnel: w285 -> [_ w308 _ w345 w348 w351 w354]
      tunnel: w278 -> [_ w307 w340 w343 w349 w352 w355]
      tunnel: w283 -> [_ _ _ w344 w347 _ _]
      tunnel: [FALSE ("error") w306 w324 w341 w346 w350 w353] -> w282
      frame "Faux", Default {
      }
      frame "Read" {
        n279 = case shown="0, Par défaut" w308 {
          selector: w308 -> [_ w313 w322]
          tunnel: w307 -> [_ w314 w323]
          tunnel: [FALSE ("Error") w310 w317] -> w306
          frame 0, Default {
          }
          frame 1 {
            n280 = call "ESP301_Read_Position.vi"("axisNumber"=w313, "COM_PORT"=w314) -> ("MD"=w311:bool, "Motor_status"=w315:bool, "Position"=w316:dbl, "Error"=w310:bool)  [unwired: 5 in, 1 out]
            n281 = Not(x=w311) -> (.not. x?=w312:bool)
            n282 = local write "ESP301_ROT_POS"(w316) -> ()
            n283 = local write "ESP301_ROT_MO"(w315) -> ()
            n284 = local write "ROT_mouvement"(w312) -> ()
          }
          frame 2 {
            n285 = call "ESP301_Read_Position.vi"("axisNumber"=w322, "COM_PORT"=w323) -> ("MD"=w318:bool, "Motor_status"=w320:bool, "Position"=w321:dbl, "Error"=w317:bool)  [unwired: 5 in, 1 out]
            n286 = Not(x=w318) -> (.not. x?=w319:bool)
            n287 = local write "ESP301_BRAS_POS"(w321) -> ()
            n288 = local write "BRAS _mouvement"(w319) -> ()
            n289 = local write "ESP301_BRAS_MO"(w320) -> ()
          }
        }
      }
      frame "Read2" {
        n290 = call "ESP301_Read_Double_Position.vi"("COM_PORT"=w340) -> ("MD 2"=w334:bool, "errstring 6"=w331:string, "errstring 3"=w332:string, "MD"=w336:bool, "Motor_status 2"=w333:bool, "Motor_status"=w338:bool, "Position 2"=w327:dbl, "Position"=w339:dbl, "error"=w324:bool)  [unwired: 2 in]
        n291 = Not(x=w336) -> (.not. x?=w337:bool)
        n292 = Not(x=w334) -> (.not. x?=w335:bool)
        n293 = local write "ESP301_ROT_POS"(w339) -> ()
        n294 = local write "ESP301_ROT_MO"(w338) -> ()
        n295 = local write "ROT_mouvement"(w337) -> ()
        n296 = local write "BRAS _mouvement"(w335) -> ()
        n297 = local write "ESP301_BRAS_MO"(w333) -> ()
        n298 = local write "ESP301_BRAS_POS"(w327) -> ()
        n299 = Empty String/Path?(string/path=w332) -> (empty?=w330:bool)
        n300 = Empty String/Path?(string/path=w331) -> (empty?=w329:bool)
        n301 = And(x=w330, y=w329) -> (x .and. y?=w328:bool)
        n302 = local write "Comm"(w328) -> ()
        n303 = Greater?(x=w327, y=38.0) -> (0:w325:bool)
        n304 = local write "BRAS_OUT"(w325) -> ()
      }
      frame "Home" {
        n305 = call "ESP301_Home.vi"("mode"=2, "homePresetPosition"=w344, "axisNumber"=w345, "COM_PORT"=w343) -> ("error"=w341:bool)  [unwired: 7 in]
      }
      frame "PA" {
        n306 = call "ESP301_PA.vi"("position"=w347, "axisNumber"=w348, "COM_PORT"=w349) -> ("error"=w346:bool)  [unwired: 7 in, 1 out]
      }
      frame "MF" {
        n307 = call "ESP301_MF.vi"("axisNumber"=w351, "COM_PORT"=w352) -> ("error"=w350:bool)  [unwired: 8 in, 1 out]
      }
      frame "STOP" {
        n308 = call "ESP301_STOP.vi"("axisNumber"=w354, "COM_PORT"=w355) -> ("Error"=w353:bool)  [unwired: 8 in, 1 out]
      }
    }
    n309 = local read "stop"() -> (w284:bool)
    n310 = case shown="Vrai" w282 {
      frame False {
      }
      frame True {
        w303 = u16 6 items=["Error"=6, "Stop"=5, "Out"=4, "In"=3, "Set"=2, "Home"=1, "Standby"=0] ("BRAS_state")
        w304 = u16 6 items=["Error"=6, "Stop"=4, "Nord"=3, "Set"=2, "Home"=1, "Standby"=0] ("ROT_state")
        n311 = local write "ROT_state"(w304) -> ()
        n312 = local write "BRAS_state"(w303) -> ()
      }
    }
  }
  n313 = disable-structure shown="Activé" {
    frame Enabled {
      n314 = while {
        stop <- "stop" stop-if-true
        n315 = local read "ROT_state"() -> (w356:u16)
        n316 = Wait (ms)(milliseconds to wait=u32 1000 ("attente (ms)")) -> ()  [unwired: 1 out]
        n317 = case shown="0, Par défaut" w356 {
          frame 0, Default {
            n318 = Bundle("a", 0, 0.0) -> (w361:cluster{string, i32, dbl})  [unwired: 1 in]
            n319 = Obtain Queue(name (unnamed)="ESP301" ("nom (aucun)"), element data type=w361) -> (queue out=w360:refnum<queue>)  [unwired: 3 in, 2 out]
            n320 = Bundle("Read2", 1, 0.0) -> (w366:cluster{string, i32, dbl})  [unwired: 1 in]
            n321 = Enqueue Element(queue=w360, element=w366) -> (queue out=w359:refnum<queue>)  [unwired: 2 in, 2 out]
            n322 = Release Queue(queue=w359) -> ()  [unwired: 2 in, 3 out]
          }
          frame 6 {
            n323 = Bundle("a", 0, 0.0) -> (w374:cluster{string, i32, dbl})  [unwired: 1 in]
            n324 = Obtain Queue(name (unnamed)="ESP301" ("nom (aucun)"), element data type=w374) -> (queue out=w373:refnum<queue>, error out=w370:errorcluster)  [unwired: 3 in, 1 out]
            n325 = Flush Queue(queue=w373, error in (no error)=w370) -> (queue out=w372:refnum<queue>, error out=w371:errorcluster)  [unwired: 1 out]
            n326 = Release Queue(queue=w372, error in (no error)=w371) -> ()  [unwired: 1 in, 3 out]
          }
        }
      }
    }
    frame Disabled {
    }
  }
  n327 = while {
    stop <- w381 stop-if-true
    n328 = local read "SONDE_IN"() -> (w379:bool)
    n329 = Wait (ms)(milliseconds to wait=u32 200 ("attente (ms)")) -> ()  [unwired: 1 out]
    n330 = case shown="Vrai" w379 {
      frame True {
        w382 = T1."Disabled and Grayed Out" ("Désactivé")
        n331 = local read "BRAS_state"() -> (w384:u16)
        n332 = property on="ESP301_BRAS_IN" class="Bool (strict)"("DisabledEnum"=w382) -> ()  [unwired: 2 in, 2 out]
        n333 = property on="ESP301_BRAS_HOME" class="Bool (strict)"("DisabledEnum"=w382) -> ()  [unwired: 2 in, 2 out]
        n334 = property on="ESP301_BRAS_SET" class="Bool (strict)"("DisabledEnum"=w382) -> ()  [unwired: 2 in, 2 out]
        n335 = property on="ESP301_BRAS_OUT" class="Bool (strict)"("DisabledEnum"=w382) -> ()  [unwired: 2 in, 2 out]
        n336 = Not Equal To 0?(x=w384) -> (x != 0?=w383:bool)
        n337 = case shown="Vrai" w383 {
          frame False {
          }
          frame True {
            w385 = u16 5 items=["Stop"=5, "Out"=4, "In"=3, "Set"=2, "Home"=1, "Standby"=0] ("BRAS_state")
            n338 = local write "BRAS_state"(w385) -> ()
          }
        }
      }
      frame False {
        n339 = local read "BRAS_state"() -> (w387:u16)
        n340 = Equal To 0?(x=w387) -> (x = 0?=w386:bool)
        n341 = case shown="Vrai" w386 {
          frame True {
            w388 = T1."Enabled" ("Désactivé")
            n342 = property on="ESP301_BRAS_IN" class="Bool (strict)"("DisabledEnum"=w388) -> ()  [unwired: 2 in, 2 out]
            n343 = property on="ESP301_BRAS_HOME" class="Bool (strict)"("DisabledEnum"=w388) -> ()  [unwired: 2 in, 2 out]
            n344 = property on="ESP301_BRAS_SET" class="Bool (strict)"("DisabledEnum"=w388) -> ()  [unwired: 2 in, 2 out]
            n345 = property on="ESP301_BRAS_OUT" class="Bool (strict)"("DisabledEnum"=w388) -> ()  [unwired: 2 in, 2 out]
          }
          frame False {
          }
        }
      }
    }
    n346 = local read "stop"() -> (w381:bool)
  }
  "Comm" <- FALSE ("Comm")
  "BRAS_OUT" <- FALSE ("BRAS_OUT")
